vi "trash_Write Wrapper for FIFO Type Support.vi"(8 "error in (no error)":errorcluster, 11 "CIF_CIPC_Fifo_U8 in":refnum<class "CIF_CIPC_Fifo_U8.lvclass">) -> (0 "error out":errorcluster)   [LabVIEW 2021]
uses:
  CIF_CIPC_Fifo_U8.lvclass
  D:/dev/Packages/CIF_Channels_Core/src/CIPC_Channels/CIF_CIPC_Chan/CIF_CIPC_Chn.lvclass
  CIF_CIPC_Chan/CIF_CIPC_Chn.lvclass/CIF_CIPC_Chn.ctl
  CIF_CIPC_Chan/Accessors/Read Buffer Type.vi
  <vilib>/CIF Foundation/CIF CIPC/SubVIs/Wait For N Elements Available.vi
  <vilib>/CIF Foundation/CIF CIPC/SubVIs/Get Element Read Position.vi
  <vilib>/CIF Foundation/CIF CIPC/SubVIs/Check Error.vi
  <vilib>/CIF Foundation/CIF CIPC/SubVIs/Get dll Path.vi
  <vilib>/CIF Foundation/CIF CIPC/SubVIs/Set Element Read Position.vi
  Write Wrapper for FIFO Type Support.vi/5d919423-ef01-4d49-a0b2-6d9051ec7dc1.vi/331f6ecb-7ec4-4931-b93d-4fbd8d66a851.vi
  Write Wrapper for FIFO Type Support.vi/5d919423-ef01-4d49-a0b2-6d9051ec7dc1.vi/5ce0d4cf-f921-42ba-b14c-c90f7f7611e4.vi
  <vilib>/CIF Foundation/CIF CIPC/SubVIs/Notify Of New Write.vi
  <vilib>/CIF Foundation/CIF CIPC/SubVIs/Get Element Write Position.vi
  <vilib>/Utility/error.llb/Trim Whitespace.vi
  <vilib>/Utility/error.llb/Error Cluster From Error Code.vi
  <vilib>/CIF Foundation/CIF CIPC/SubVIs/Get Element Info Variant.vi
  CIF_CIPC_Fifo_U8.lvclass/CIF_CIPC_Fifo_U8.ctl
  CIF_CIPC_Chan/CIF_CIPC_Chn.lvclass
  bf61965d-de10-4d44-a0c8-f163c280b891.vi
  D:/dev/Packages/CIF_Channels_Core/src/CIFChannels/CIFChannels.lvclass
  D:/dev/Packages/CIF_Channels_Core/src/CIPC_Channels/FIFO_U8/CIF_CIPC_Fifo_U8.lvclass
panel:
  in  "Timeout (ms)":i32
  out "timed out?":bool
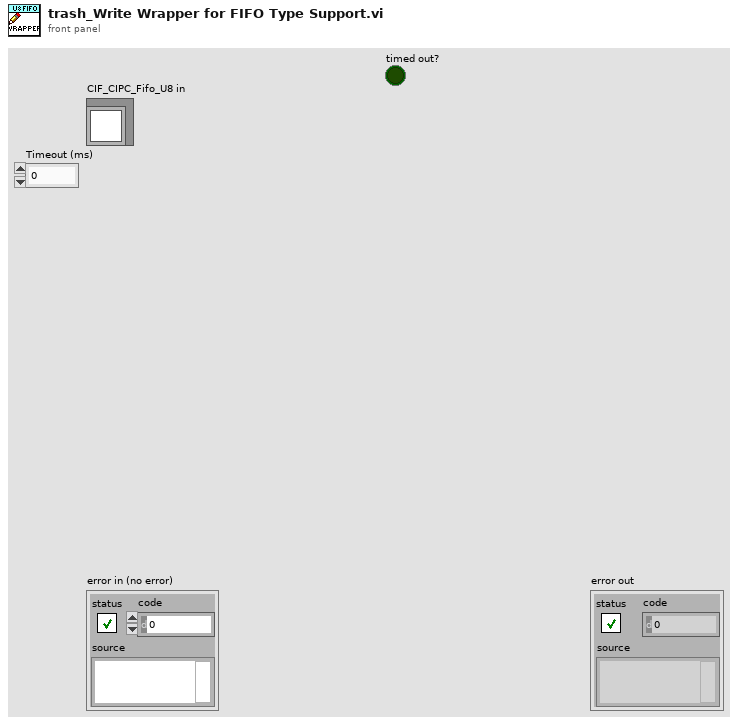
[diagram p1: front panel]
types:
  T1 = typedef "CIF_CIPC_Chn.lvclass/Buffer Type.ctl" = enum16{"FIFO", "Backpressure FIFO"}
  T2 = typedef "CIF_CIPC_Chn.lvclass/Buffer Configuration Data.ctl" = cluster{"Total Size":u32, "Read Size":u32, "Read Offset":u32, "CIPC BP References":T3, "Override CIPC Name":string, "Encoder Data":string}
  T3 = typedef "CIF_NI_CIPC.lvlib/Backpressure References.ctl" = cluster{"CIPC Reference":u64, "CIPC BP Reference":u64}
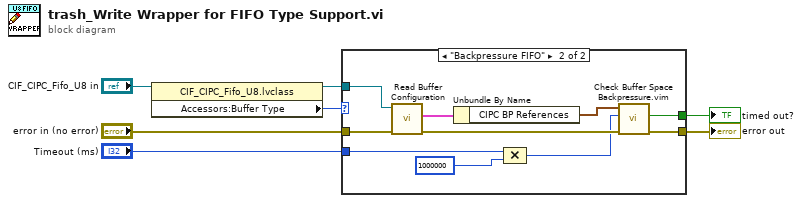
[diagram p0: block diagram]
diagram:
  n1 = property class="CIF_CIPC_Fifo_U8.lvclass"(reference="CIF_CIPC_Fifo_U8 in") -> (reference out=w4:refnum<class "CIF_CIPC_Fifo_U8.lvclass">, "Accessors:Buffer Type"=w3:T1)  [unwired: 1 in, 1 out]
  n2 = case shown="\"Backpressure FIFO\"" w3 {
    tunnel: [w8 w9] -> w7
    tunnel: "error in (no error)" -> [w8 w17]
    tunnel: w4 -> [_ w18]
    tunnel: [_ w13] -> w2
    tunnel: "Timeout (ms)" -> [_ w12]
    frame "FIFO" {
    }
    frame "Backpressure FIFO" {
      n3 = call "Read Buffer Configuration.vi"("error in (no error)"=w17, "CIF_CIPC_Chn in"=w18) -> ("error out"=w14:errorcluster, "Buffer Configuration"=w16:T2)  [unwired: 7 in, 1 out]
      n4 = Unbundle By Name(w16) -> ("CIPC BP References"=w15:T3)
      n5 = Compound Arithmetic op=MULTIPLY(w12, 1000000 ("value")) -> (w10:i32)
      n6 = call "Check Buffer Space Backpressure.vim"("error in (no error)"=w14, "Timeout (ns)"=w10, "CIPC BP References in"=w15) -> ("error out"=w9:errorcluster, "Timeout"=w13:bool)  [unwired: 6 in, 1 out]
    }
  }
  "error out" <- w7
  "timed out?" <- w2
